vi "Populate Manufacturer Specific Objects.vi"(8 "error in":errorcluster, 11 "UI Actor in":refnum<class "UI Actor.lvclass">) -> (0 "error out":errorcluster)   [LabVIEW 2020, in "UI Actor.lvlib" / "UI Actor.lvclass"]
uses:
  UI Actor.lvclass
  UI Actor.lvclass/UI Actor.ctl
  Electronic Datasheet/Electronic Datasheet.lvclass
  Core/OD Entry/OD Entry.lvclass
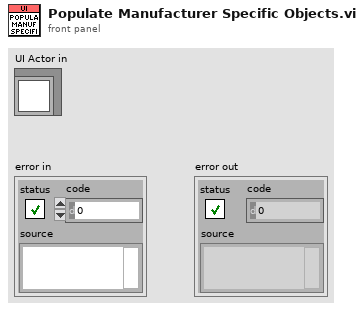
[diagram p1: front panel]
types:
  T1 = map{path, refnum<class "Electronic Datasheet.lvclass">}
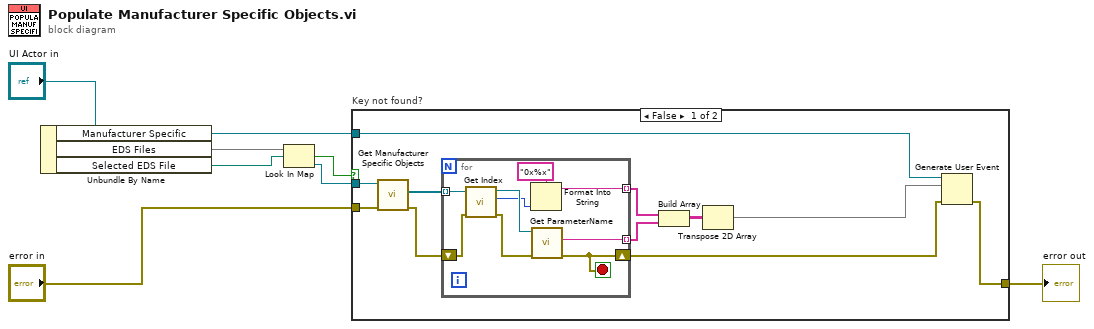
[diagram p0: block diagram]
diagram:
  n1 = Unbundle By Name("UI Actor in") -> ("Manufacturer Specific"=w1:refnum<user-event>, "EDS Files"=w8:T1, "Selected EDS File"=w7:path)
  n2 = Look In Map(map=w8, key=w7) -> (key not found?=w6:bool, value=w5:refnum<class "Electronic Datasheet.lvclass">)  [unwired: 1 in]
  n3 = case "Key not found?" shown="False" w6 {
    tunnel: w5 -> [w19 _]
    tunnel: "error in" -> [w18 w29]
    tunnel: [w10 w29] -> w2
    tunnel: w1 -> [w9 _]
    frame False {
      n4 = call "Get Manufacturer Specific Objects.vi"("error in"=w18, "reference in"=w19) -> ("error out"=w16:errorcluster, "Entries"=w17:refnum<class "OD Entry.lvclass">[])  [unwired: 7 in, 1 out]
      n5 = for {
        tunnel: w17 -> [w28] mode=indexing
        tunnel: [w25] -> w12 mode=indexing
        shift-right: [w20] -> w11
        shift-left: w16 -> [w24]
        tunnel: [w21] -> w13 mode=indexing
        stop <- w20 stop-if-true
        n6 = call "Get Index.vi"("Error In"=w24, "reference in"=w28) -> ("Error Out"=w26:errorcluster, "Index"=w23:u16, "reference out"=w27:refnum<class "OD Entry.lvclass">)  [unwired: 7 in]
        n7 = Format Into String(format string="0x%x", w23) -> (resulting string=w21:string)  [unwired: 2 in, 1 out]
        n8 = call "Get ParameterName.vi"("Error In"=w26, "reference in"=w27) -> ("Error Out"=w20:errorcluster, "ParameterName"=w25:string)  [unwired: 7 in, 1 out]
      }
      n9 = Build Array(w13, w12) -> (w14:string[][])
      n10 = Transpose 2D Array(2D array=w14) -> (transposed array=w15:string[][])
      n11 = Generate User Event(user event=w9, event data cluster=w15, error in=w11) -> (error out=w10:errorcluster)  [unwired: 1 in, 1 out]
    }
    frame True {
    }
  }
  "error out" <- w2
